vi "WPI_IMU_ADIS16460_ReadRegister.vi"(8 "error in (no error)":errorcluster, 10 "ADIS16460 Register":T1=86 items=["PROD_ID"=86, "GLOB_CMD"=62, "DEC_RATE"=54, "FLTR_CTRL"=56, "MSC_CTRL"=50], 11 "SPIDevRef in":T2) -> (0 "error out":errorcluster, 2 "Register Value":u16, 3 "SPIDevRef out":T2)   [LabVIEW 2015, in "FRC ADIS16460.lvlib"]
uses:
  FRC ADIS16460.lvlib
  <vilib>/Rock Robotics/WPI/SPI/WPI_SPIDevRef.ctl
  <vilib>/Rock Robotics/SystemInterfaces/spilib/spi_bus.ctl
  WPI_IMU_ADIS16460_Registers.ctl
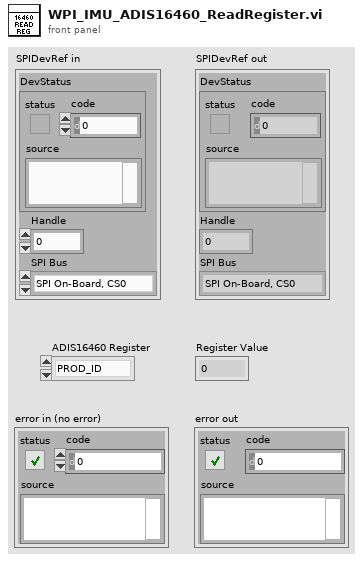
[diagram p1: front panel]
types:
  T1 = typedef "FRC ADIS16460.lvlib/WPI_IMU_ADIS16460_Registers.ctl" = u8
  T2 = typedef "WPI_SPIDevRef.ctl" = cluster{"DevStatus":errorcluster, "Handle":i32, "SPI Bus":T3}
  T3 = typedef "spi_bus.ctl" = enum16{"SPI On-Board, CS0", "SPI On-Board, CS1", "SPI On-Board, CS2", "SPI On-Board, CS3", "SPI MXP", "Invalid"}
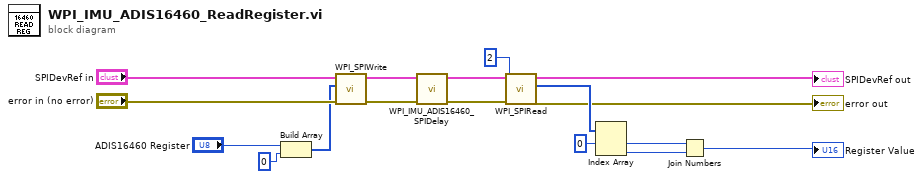
[diagram p0: block diagram]
diagram:
  n1 = Build Array("ADIS16460 Register", u8 0 ("element")) -> (w8:T1[])
  n2 = call <vilib>:"WPI_SPIWrite.vi"("error in (no error)"="error in (no error)", "Data To Send"=w8, "SPIDevRef"="SPIDevRef in") -> ("error out"=w4:errorcluster, "SPIDevRef"=w3:T2)  [unwired: 7 out]
  n3 = call "WPI_IMU_ADIS16460_SPIDelay.vi"("error in"=w4, "SPIDevRef in"=w3) -> ("error out"=w1:errorcluster, "SPIDevRef out"=w2:T2)  [unwired: 8 in]
  n4 = call <vilib>:"WPI_SPIRead.vi"("error in (no error)"=w1, "Num to Read"=2, "SPIDevRef"=w2) -> ("error out"=→"error out":errorcluster, "Received Data"=w12:u8[], "SPIDevRef"=→"SPIDevRef out":T2)  [unwired: 6 in]
  n5 = Index Array(array=w12, index #1=0 ("index")) -> (element #1=w7:u8, element #2=w6:u8)  [unwired: 1 in]
  n6 = Join Numbers(hi=w7, lo=w6) -> ((hi.lo)=→"Register Value":u16)
